vi "Gevt-ThreadQueueName.vi"() -> (1 "ThreadQueueName":string="_CSM_GEvt_BackgroundThread")   [LabVIEW 2017, in "Communicable State Machine.lvlib"]
doc: "-- <b>Indicators</b> --\n- <b>ThreadQueueName</b>:"
uses:
  Communicable State Machine.lvlib
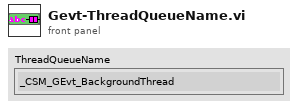
[diagram p1: front panel]
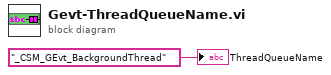
[diagram p0: block diagram]
diagram:
  "ThreadQueueName" <- "_CSM_GEvt_BackgroundThread" ("name (unnamed)")
